vi "价格公式.vi"(8 "error in (no error)":errorcluster caption="错误输入（无错误）", 10 "基础价格":dbl, 11 "大杯 输入":refnum<class "大杯.lvclass">) -> (0 "error out":errorcluster caption="错误输出", 2 "价格":dbl, 3 "大杯 输出":refnum<class "大杯.lvclass">)   [LabVIEW 2016, in "大杯.lvclass"]
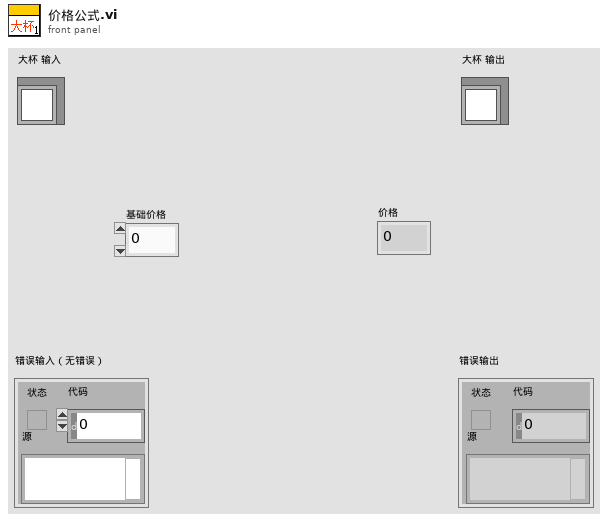
[diagram p1: front panel]
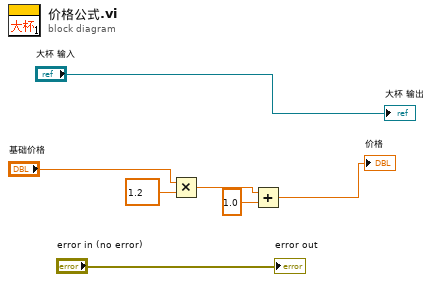
[diagram p0: block diagram]
diagram:
  n1 = Multiply(x="基础价格", y=1.2) -> (x*y=w3:dbl)
  n2 = Add(x=w3, y=1.0) -> (x+y=→"价格":dbl)
  "error out" <- "error in (no error)"
  "大杯 输出" <- "大杯 输入"
